vi "Velocity Converter- Speed-Direction to X-Y.vi"(10 "Speed":dbl, 11 "Heading":T2 format="%05.1f") -> (3 "Robot Velocity Out":T1)   [LabVIEW 2011]
doc: "Converts velocity in the Direction/Speed format (as defined in the appropriate Typedef) to X/Y velocity, which is the standard type within our architecture."
uses:
  2 Typedefs/heading.ctl
  2 Typedefs/robot velocity.ctl
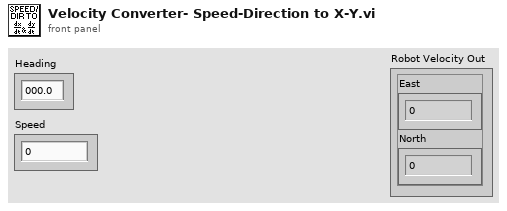
[diagram p1: front panel]
types:
  T1 = typedef "robot velocity.ctl" = cluster{"East":dbl, "North":dbl}
  T2 = typedef "heading.ctl" = dbl
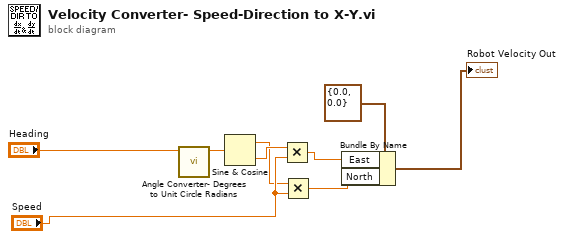
[diagram p0: block diagram]
diagram:
  n1 = call "Angle Converter- Degrees to Unit Circle Radians.vi"("Angle in \nHeading \nFormat"="Heading") -> ("Angle in \nUnit Circle\nRadians"=w6:dbl)  [unwired: 10 in]
  n2 = Sine & Cosine(0:w6) -> (1:w4:dbl, 2:w5:dbl)
  n3 = Multiply(x=w5, y="Speed") -> (x*y=w8:dbl)
  n4 = Multiply(x=w4, y="Speed") -> (x*y=w9:dbl)
  n5 = Bundle By Name(cluster=T1 {"East"=0.0, "North"=0.0} ("Robot Velocity"), "East"=w8, "North"=w9) -> (→"Robot Velocity Out":T1)
